vi "Validate Enum Strings.vi"(8 "error in":errorcluster, 11 "measurement plugin service in":refnum<class "Measurement Plugin Service.lvclass">) -> (0 "error out":errorcluster, 3 "measurement plugin service out":refnum<class "Measurement Plugin Service.lvclass">)   [LabVIEW 2020, in "MeasurementLink Measurement Server.lvlib"]
uses:
  MeasurementLink Measurement Server.lvlib
  Error Strings Global Internal.vi
  Measurement Plugin Service/Measurement Plugin Service.lvclass
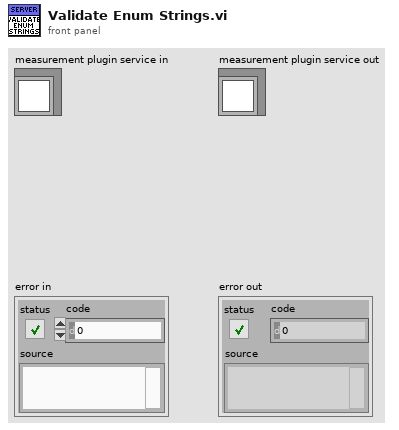
[diagram p1: front panel]
types:
  T1 = typedef "MeasurementLink Measurement Server.lvlib/Measurement Plugin Service.lvclass/Plugin Paths.ctl" = cluster{"Get Measurement Details VI Path":path, "Get Type Specializations VI Path":path, "Get UI Details VI Path":path, "Measurement Logic VI Path":path, "Measurement Configuration CTL Path":path, "Measurement Results CTL Path":path}
  T2 = cluster{"Enum reference out":refnum<vi>, "Label.Text":string}[]
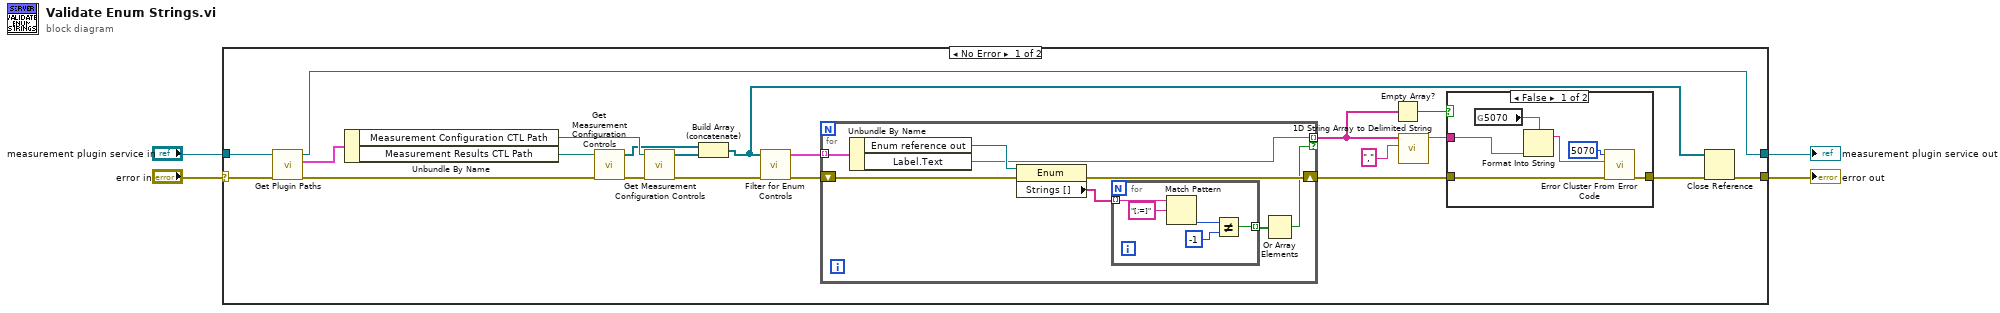
[diagram p0: block diagram]
diagram:
  n1 = case shown="No Error" "error in" {
    selector: "error in" -> [w24 w47]
    tunnel: "measurement plugin service in" -> [w25 w46]
    tunnel: [w6 w47] -> w2
    tunnel: [w13 w46] -> w1
    frame No Error {
      n2 = call-dynamic "Get Plugin Paths.vi"("error in (no error)"=w24, "MeasurementPluginService in"=w25) -> ("error out"=w23:errorcluster, "Plugin Paths"=w22:T1, "MeasurementPluginService out"=w13:refnum<class "Measurement Plugin Service.lvclass">)  [unwired: 7 in]
      n3 = Unbundle By Name(w22) -> ("Measurement Configuration CTL Path"=w19:path, "Measurement Results CTL Path"=w20:path)
      n4 = call "Get Measurement Configuration Controls.vi"("error in (no error)"=w23, "measurement configuration control path"=w20) -> ("error out"=w21:errorcluster, "Controls[]"=w16:refnum<vi>[])  [unwired: 7 in]
      n5 = call "Get Measurement Configuration Controls.vi"("error in (no error)"=w21, "measurement configuration control path"=w19) -> ("error out"=w18:errorcluster, "Controls[]"=w17:refnum<vi>[])  [unwired: 7 in]
      n6 = Build Array (concatenate)(w16, w17) -> (w5:refnum<vi>[])
      n7 = call "Filter for Enum Controls.vi"("error in (no error)"=w18, "Controls[]"=w5) -> ("error out"=w14:errorcluster, "Enum Controls and Labels[]"=w15:T2)  [unwired: 8 in]
      n8 = for {
        tunnel: w15 -> [w33] mode=indexing
        shift-right: [w32] -> w8
        shift-left: w14 -> [w30]
        tunnel: [w28] -> w9 mode=indexing if=w26
        n9 = Unbundle By Name(w33) -> ("Enum reference out"=w31:refnum<vi>, "Label.Text"=w28:string)
        n10 = property class="Enum"(reference=w31, error in=w30) -> (error out=w32:errorcluster, "Strings []"=w29:string[])  [unwired: 1 out]
        n11 = for {
          tunnel: w29 -> [w37] mode=indexing
          tunnel: [w34] -> w27 mode=indexing
          n12 = Match Pattern(string=w37, regular expression="[;=]" ("string")) -> (offset past match=w36:i32)  [unwired: 1 in, 3 out]
          n13 = Not Equal?(x=w36, y=-1) -> (x != y?=w34:bool)
        }
        n14 = Or Array Elements(Boolean array=w27) -> (logical OR=w26:bool)
      }
      n15 = Empty Array?(array=w9) -> (empty?=w11:bool)
      n16 = call <vilib>:"1D String Array to Delimited String.vi"("delimiter"=",", "string array"=w9) -> ("delimited string"=w10:string)  [unwired: 9 in]
      n17 = case shown="False" w11 {
        tunnel: w10 -> [w43 _]
        tunnel: w8 -> [w39 w45]
        tunnel: [w40 w45] -> w7
        frame False {
          n18 = global read "Error Strings Global Internal.vi" "5070"() -> (w41:string)
          n19 = Format Into String(format string=w41, w43) -> (resulting string=w42:string)  [unwired: 2 in, 1 out]
          n20 = call <vilib>:"Error Cluster From Error Code.vi"("error in (no error)"=w39, "error message (\"\")"=w42, "error code (0)"=5070) -> ("error out"=w40:errorcluster)  [unwired: 6 in]
        }
        frame True {
        }
      }
      n21 = Close Reference(reference=w5, error in (no error)=w7) -> (error out=w6:errorcluster)
    }
    frame Error {
    }
  }
  "measurement plugin service out" <- w1
  "error out" <- w2
